vi "downloadFile.vi"(6 "error in (no error)":errorcluster, 7 "File Reference":refnum<k24>, 8 "Local Path":path, 9 "Google Drive Service Ref":refnum<k24>) -> (0 "error out":errorcluster)   [LabVIEW 2018, in "GDrive.lvlib"]
doc: "This VI takes in the authentication from the Google Drive Service Reference and a file reference. Based on those inputs, this VI will download the corresponding file to the specified path."
uses:
  GDrive.lvlib
  Y:/UCLA Google Drive/Xavier's Retina MBP/LabVIEW/GDrive/Dependencies/Google.Apis.Drive.v3.dll
  Dependencies/Google.Apis.Drive.v3.dll
  <vilib>/Utility/config.llb/Read Key (String).vi
  <vilib>/Utility/config.llb/NI_LVConfig.lvlib
panel:
  # "The user must provide a path for the file to be\ndownloaded to."
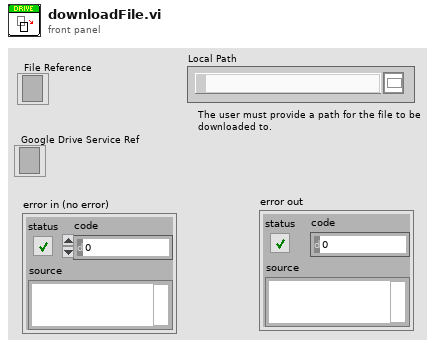
[diagram p1: front panel]
types:
  T1 = typedef "NI_LVConfig.lvlib/Config Data RefNum.ctl" = refnum<k1>
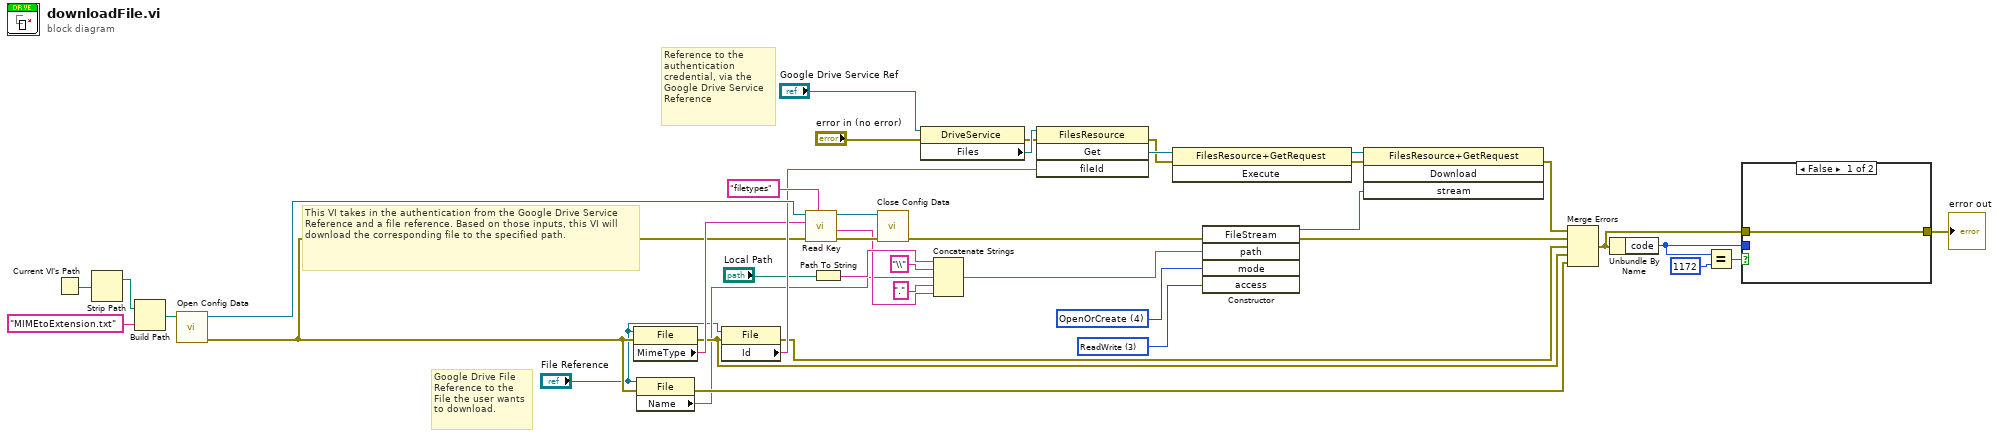
[diagram p0: block diagram]
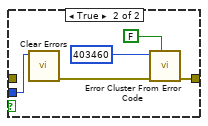
[diagram p2: hidden frame]
diagram:
  w40 = 3 items=["Read"=1, "Write"=2, "ReadWrite"=3] ("access")
  w39 = 4 items=["CreateNew"=1, "Create"=2, "Open"=3, "OpenOrCreate"=4, "Truncate"=5, "Append"=6] ("mode")
  # "Google Drive File\nReference to the \nFile the user wants\nto download."
  # "Reference to the authentication credential, via the Google Drive Service Reference"
  # "This VI takes in the authentication from the Google Drive Service Reference and a file reference. Based on those inputs, this VI will download the corresponding file to the specified path."
  n1 = Current VI's Path() -> (path=w10:path)
  n2 = Strip Path(path=w10) -> (stripped path=w11:path)  [unwired: 1 out]
  n3 = Build Path(base path=w11, name or relative path="MIMEtoExtension.txt") -> (appended path=w26:path)
  n4 = call <vilib>:"Open Config Data.vi"("configuration file path"=w26) -> ("error out"=w9:errorcluster, "refnum"=w30:T1)  [unwired: 8 in, 1 out]
  n5 = property class="File"(reference="File Reference", error in=w9) -> (error out=w8:errorcluster, "MimeType"=w20:string)  [unwired: 1 out]
  n6 = property class="File"(reference="File Reference", error in=w9) -> (error out=w13:errorcluster, "Name"=w3:string)  [unwired: 1 out]
  n7 = property class="File"(reference="File Reference", error in=w8) -> (error out=w14:errorcluster, "Id"=w21:string)  [unwired: 1 out]
  n8 = call-poly <vilib>:"Read Key.vi"("section"="filetypes", "error in (no error)"=w9, "key"=w20, "refnum"=w30) -> ("error out"=w27:errorcluster, "value"=w5:string, "refnum out"=w28:T1)  [unwired: 4 in, 1 out]
  n9 = Path To String(path="Local Path") -> (string=w6:string)
  n10 = call <vilib>:"Close Config Data.vi"("error in (no error)"=w27, "refnum"=w28) -> ("error out"=w24:errorcluster)  [unwired: 8 in, 1 out]
  n11 = property class="DriveService"(reference="Google Drive Service Ref", error in="error in (no error)") -> (error out=w34:errorcluster, "Files"=w37:refnum<k24>)  [unwired: 1 out]
  n12 = Concatenate Strings(w6, "\\" ("string"), w3, ".", w5) -> (w31:string)
  n13 = invoke class="FilesResource" method="Get"(reference=w37, error in=w34, "fileId"=w21) -> (error out=w33:errorcluster, "Get"=w36:refnum<k24>)  [unwired: 1 in, 2 out]
  n14 = invoke class="FilesResource+GetRequest" method="Execute"(reference=w36, error in=w33) -> (reference out=w35:refnum<k24>, error out=w32:errorcluster)  [unwired: 1 in, 1 out]
  n15 = constructor class="FileStream"(error in=w24, "path"=w31, "mode"=w39, "access"=w40) -> (reference out=w38:refnum<k24>, error out=w22:errorcluster)  [unwired: 2 in, 4 out]
  n16 = invoke class="FilesResource+GetRequest" method="Download"(reference=w35, error in=w32, "stream"=w38) -> (error out=w23:errorcluster)  [unwired: 1 in, 3 out]
  n17 = Merge Errors(w23, w22, w14, w8, w13) -> (w16:errorcluster)
  n18 = Unbundle By Name(w16) -> ("code"=w17:i32)
  n19 = Equal?(x=w17, y=1172) -> (x = y?=w18:bool)
  n20 = case shown="False" w18 {
    tunnel: w17 -> [_ w47]
    tunnel: [w42 w46] -> w12
    tunnel: w16 -> [w42 _]
    frame False {
    }
    frame True {
      n21 = call <vilib>:"Clear Errors.vi"("specific error code to clear (0: all)"=w47) -> ("error out"=w44:errorcluster)  [unwired: 5 in, 1 out]
      n22 = call <vilib>:"Error Cluster From Error Code.vi"("show call chain? (False)"=FALSE, "error in (no error)"=w44, "error code (0)"=403460) -> ("error out"=w46:errorcluster)  [unwired: 6 in]
    }
  }
  "error out" <- w12
